vi "TakeVData_CO.vi"(0 "Sensor":u16(ring)=1 items=["No1"=1, "No 2"=2, "No 3"=3, "No 4"=4], 2 "Measurement wait time (ms)":dbl=100.0, 3 "Setpoint temperature (K)":dbl=21.72 format="%.3f", 4 "Allowable deviation (K)":dbl=0.002 format="%.4f", 5 "Number of voltage measurements\nbetween temperature check":dbl=8.0, 6 "Temperature Controller GPIB address":string="10", 8 "DMM (to sample) GPIB address":string="17", 10 "DMM2 GPIB address":string="30", 15 "Cutoff (nV)":dbl=0.3 format="%.2f") -> (7 "Mean Temp (C)":dbl=8.900000000000008e-06 format="%.6f", 9 "Temp error (C)":dbl=8.479922812684727e-07 format="%.6f", 11 "Voltage error 2 (mV)":dbl=8.479922812684727e-07 format="%.6f", 13 "Mean Voltage 2 (mV)":dbl=8.900000000000008e-06 format="%.6f", 16 "Temperature stable?":bool=TRUE, 17 "Mean Voltage 1 (mV)":dbl=2.5123402777783724e-08 format="%_4e", 18 "Voltage error 1 (mV)":dbl=9.655250545895796e-07 format="%.6f", 19 "Number of measurements":dbl=72.0)   [LabVIEW 2014]
uses:
  <vilib>/Analysis/NI_AALBase.lvlib
panel:
  out "Current mean":dbl=2.5123402777783724e-08 format="%_4e"
  out "XY Graph":T1(graph)={"X Values"=[-1.3009003499999803e-05, -9.481650499999804e-06, -5.954297499999805e-06, -2.4269444999998053e-06, 1.1004085000001942e-06, 4.627761500000194e-06, 8.155114500000194e-06, 1.1682467500000193e-05, 1.5209820500000192e-05, 1.873717350000019e-05], "Histogram: h(x)"=[6, 7, 10, 12, 13, 7, 8, 6, 1, 2]}
  out "Waveform Chart":dbl[](graph)=[-4.220760000000091e-06, -1.0250409999999939e-05, -4.8237250000000755e-06, 5.728169999999954e-06, -1.085337500000014e-05, 0.0, 8.140034999999874e-06, -3.316314999999995e-06, 5.4266849999998635e-06, -1.447117000000003e-05, -6.029655000000045e-06, -3.617790000000126e-06, -1.5074100000000805e-06, 6.934104999999904e-06, -1.3566725000000151e-05, 9.34596500000006e-06, 2.1103800000000453e-06, 1.8088999999999345e-06, -3.0148500000009085e-07, -4.522244999999965e-06, 9.34597500000002e-06, 3.014825000000141e-06, 4.522239999999985e-06, 1.2360785000000221e-05, -1.4169710000000056e-05, 1.899344000000011e-05, -4.823729999999839e-06, 9.647459999999894e-06, 8.743010000000035e-06, 0.0, -3.014800000001108e-07, -1.4772679999999804e-05, -4.220759999999874e-06, 9.34596500000006e-06, -1.2059299999999697e-06, -1.1154869999999975e-05, 6.029649999999848e-07, 1.0250424999999879e-05, 2.0500850000000192e-05, -6.331144999999682e-06, -2.71335000000001e-06, -3.014800000001108e-07, 1.1757835000000176e-05, -8.743005000000055e-06, -1.5074150000000605e-06, 6.331139999999919e-06, -2.4118649999999194e-06, 1.2059349999999497e-06, -8.140044999999834e-06, -5.728179999999914e-06, 1.5978610000000207e-05, -8.441524999999945e-06, 1.175783999999994e-05, -1.2662294999999995e-05, 9.647459999999894e-06, 1.1154869999999975e-05, -6.934115000000081e-06, -6.02964999999768e-07, -3.01484999999874e-07, -1.2059349999999497e-06, 0.0, 1.1154869999999975e-05, -3.014830000000121e-06, -7.83855999999996e-06, 5.42669500000004e-06, -3.617795000000106e-06, -3.91927999999998e-06, -1.5074150000000605e-06, 3.014830000000121e-06, -1.175783999999994e-05, -6.934115000000081e-06, 3.01484999999874e-07]
  out "Loop No.":dbl=8.0 format="%#_4f"
  out "Current precision":dbl=0.026020456598573768 format="%_6f"
  out "Current error (mV)":dbl=9.655250545895796e-07 format="%_4e"
  in  "Precision":dbl=1000.0 format="%.2f"
  # "For high precision,\n0.15 works well."
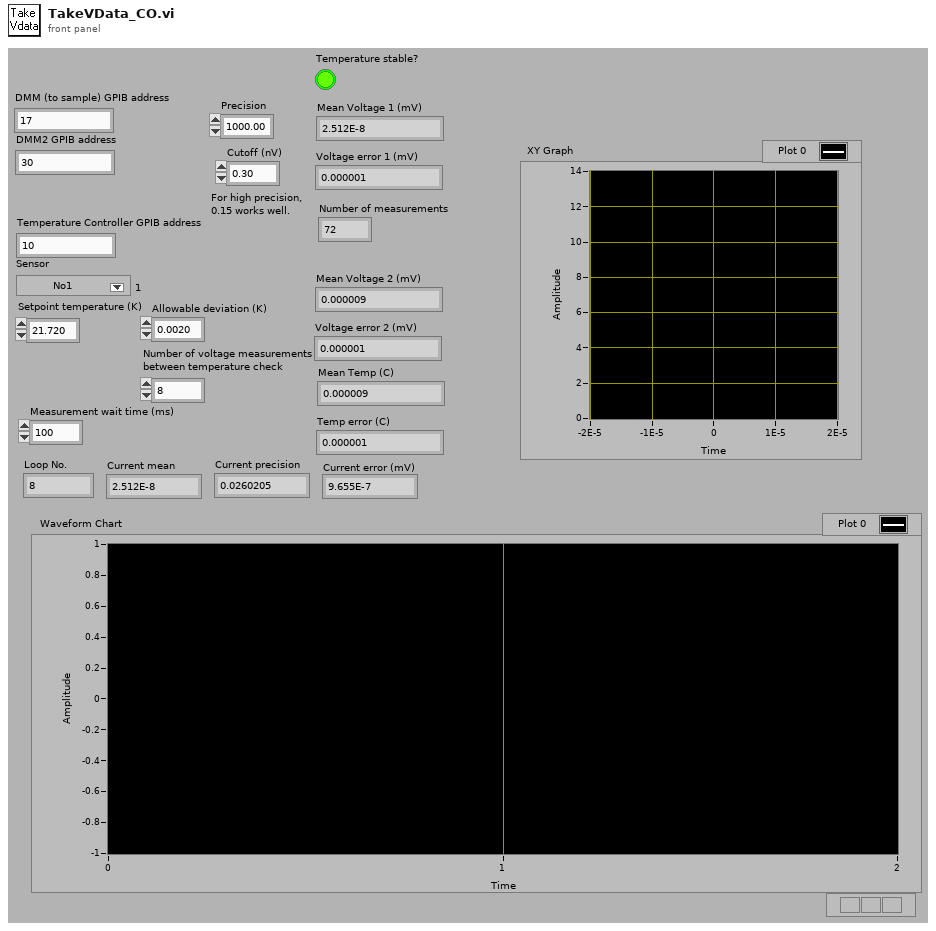
[diagram p1: front panel]
types:
  T1 = cluster{"X Values":dbl[], "Histogram: h(x)":i32[]}
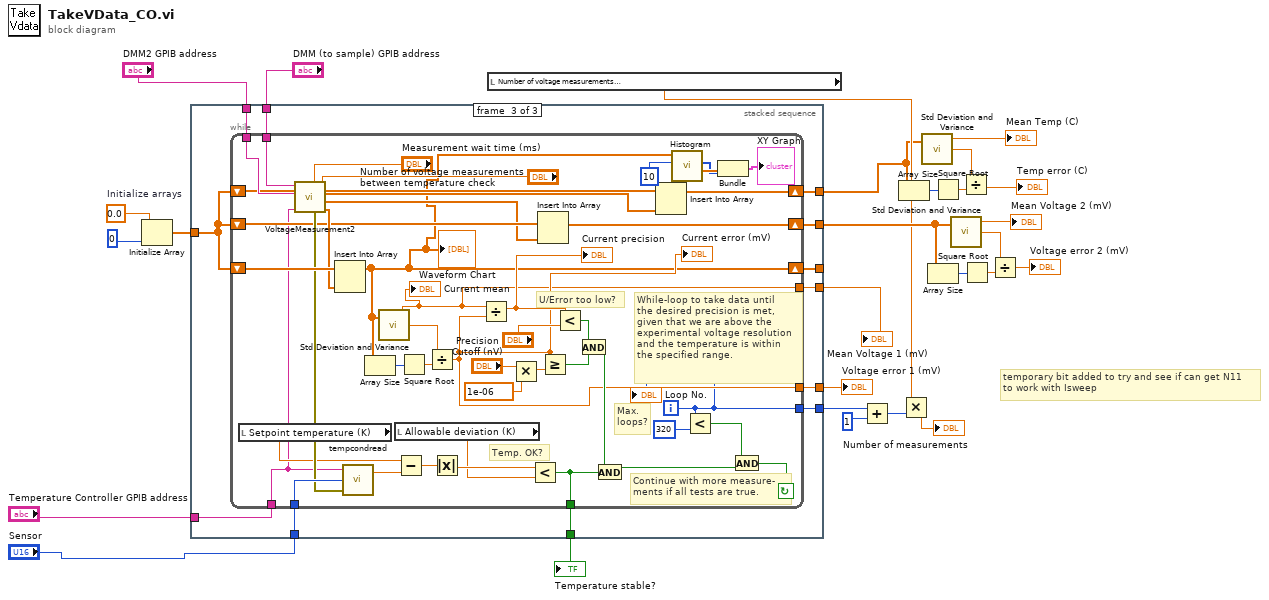
[diagram p0: block diagram]
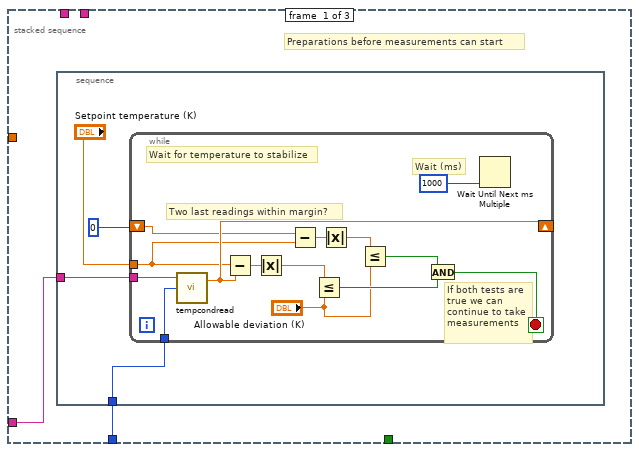
[diagram p2: hidden frame]
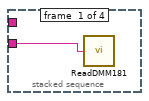
[diagram p4: hidden frame]
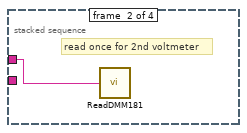
[diagram p5: hidden frame]
diagram:
  w25 = 0.0  # Initialize arrays
  # "temporary bit added to try and see if can get N11\nto work with Isweep"
  n1 = Initialize Array(w25, 0) -> (w24:dbl[])
  n2 = stacked-sequence {
    tunnel: "DMM (to sample) GPIB address" -> [_ w49 w63]
    tunnel: w24 -> [_ _ w53]
    tunnel: "Sensor" -> [w28 _ w62]
    tunnel: "Temperature Controller GPIB address" -> [w29 _ w61]
    tunnel: [_ _ w60] -> w22
    tunnel: [_ _ w59] -> _
    tunnel: [_ _ w58] -> w20
    tunnel: [_ _ w57] -> w17
    tunnel: [_ _ w56] -> w8
    tunnel: "DMM2 GPIB address" -> [_ w48 w55]
    tunnel: [_ _ w54] -> w12
    tunnel: [_ _ w52] -> w2
    frame #0 {
      # "Preparations before measurements can start"
      n3 = stacked-sequence {
        tunnel: w29 -> [w33]
        tunnel: w28 -> [w32]
        frame #0 {
          n4 = while {
            shift-left: 0 -> [w35]
            shift-right: [w37] -> _
            tunnel: w32 -> [w41]
            tunnel: w33 -> [w45]
            tunnel: "Setpoint temperature (K)" -> [w36]
            stop <- w43 stop-if-true
            # "If both tests are\ntrue we can\ncontinue to take\nmeasurements"
            # "Two last readings within margin?"
            # "Wait for temperature to stabilize"
            # "Wait (ms)"
            n5 = call "tempcondread.vi"("Ring"=w41, "GPIB Address"=w45) -> ("Temperature"=w37:dbl)  [unwired: 1 in, 1 out]
            n6 = Subtract(x=w36, y=w37) -> (x-y=w46:dbl)
            n7 = Absolute Value(x=w46) -> (abs(x)=w42:dbl)
            n8 = Subtract(x=w35, y=w36) -> (x-y=w40:dbl)
            n9 = Less Or Equal?(x=w42, y="Allowable deviation (K)") -> (x <= y?=w44:bool)
            n10 = Absolute Value(x=w40) -> (abs(x)=w39:dbl)
            n11 = Less Or Equal?(x=w39, y="Allowable deviation (K)") -> (x <= y?=w38:bool)
            n12 = And(x=w38, y=w44) -> (x .and. y?=w43:bool)
            n13 = Wait Until Next ms Multiple(millisecond multiple=1000) -> ()  [unwired: 1 out]
          }
        }
      }
    }
    frame #1 {
      n14 = stacked-sequence {
        tunnel: w49 -> [w50 _ _ _]
        tunnel: w48 -> [_ w51 _ _]
        frame #0 {
          n15 = call "ReadDMM181.vi"("DMM GPIB Address"=w50) -> ()  [unwired: 1 out]
        }
        frame #1 {
          # "read once for 2nd voltmeter"
          n16 = call "ReadDMM181.vi"("DMM GPIB Address"=w51) -> ()  [unwired: 1 out]
        }
        frame #2 {
          # "read once for 3rd voltmeter"
        }
        frame #3 {
        }
      }
    }
    frame #2 {
      n17 = while {
        shift-left: w53 -> [w79]
        shift-right: [w78] -> w52
        shift-left: w53 -> [w86]
        shift-right: [w87] -> w54
        tunnel: w55 -> [w90]
        tunnel: [w65] -> w56
        tunnel: [w72] -> w57
        tunnel: [w71] -> w58
        tunnel: [w103] -> w60
        tunnel: w61 -> [w64]
        tunnel: w62 -> [w105]
        shift-left: w53 -> [w102]
        shift-right: [w70] -> w59
        tunnel: w63 -> [w89]
        i -> [w71]
        stop <- w97 continue-if-true
        # "U/Error too low?"
        # "Max.\nloops?"
        # "Continue with more measure-\nments if all tests are true."
        # "While-loop to take data until\nthe desired precision is met,\ngiven that we are above the\nexperimental voltage resolution\nand the temperature is within\nthe specified range."
        # "Temp. OK?"
        n18 = local read "Setpoint temperature (K)"() -> (w83:dbl)
        n19 = call "VoltageMeasurement2.vi"("Number of measurements"="Number of voltage measurements\nbetween temperature check", "Measurement wait time (ms)"="Measurement wait time (ms)", "Temp Controller address"=w64, "DMM2 GPIB address"=w90, "DMM GPIB address"=w89) -> ("Voltage 1 (mV)"=w88:dbl[], "Voltage 2 (mV)"=w85:dbl[], "Voltage 3 (mV)"=w77:dbl[], "error out"=w101:errorcluster)  [unwired: 3 in]
        n20 = Insert Into Array(array=w102, new element=w88) -> (w70:dbl[])  [unwired: 1 in]
        "Waveform Chart" <- w70
        n21 = call "tempcondread.vi"("error in"=w101, "Ring"=w105, "GPIB Address"=w64) -> ("Temperature"=w106:dbl)  [unwired: 1 out]
        n22 = Array Size(array=w70) -> (size(s)=w93:i32)
        n23 = call <vilib>:"Std Deviation and Variance.vi"("X"=w70) -> ("mean"=w65:dbl, "standard deviation"=w92:dbl)  [unwired: 1 in, 1 out]
        "Current mean" <- w65
        n24 = local read "Allowable deviation (K)"() -> (w81:dbl)
        n25 = Subtract(x=w83, y=w106) -> (x-y=w107:dbl)
        n26 = Square Root(x=w93) -> (sqrt(x)=w91:dbl)
        n27 = Divide(x=w92, y=w91) -> (x/y=w72:dbl)
        "Current error (mV)" <- w72
        n28 = Absolute Value(x=w107) -> (abs(x)=w104:dbl)
        n29 = Divide(x=w65, y=w72) -> (x/y=w73:dbl)
        "Current precision" <- w73
        n30 = Multiply(x="Cutoff (nV)", y=1e-06) -> (x*y=w74:dbl)
        n31 = Less?(x=w104, y=w81) -> (x < y?=w103:bool)
        n32 = Insert Into Array(array=w86, new element=w85) -> (w87:dbl[])  [unwired: 1 in]
        n33 = Greater Or Equal?(x=w72, y=w74) -> (x >= y?=w96:bool)
        n34 = Less?(x=w73, y="Precision") -> (x < y?=w95:bool)
        n35 = And(x=w95, y=w96) -> (x .and. y?=w94:bool)
        n36 = And(x=w94, y=w103) -> (x .and. y?=w99:bool)
        n37 = Insert Into Array(array=w79, new element=w77) -> (w78:dbl[])  [unwired: 1 in]
        n38 = call <vilib>:"Histogram.vi"("intervals"=10, "X"=w70) -> ("X Values"=w67:dbl[], "Histogram: h(x)"=w66:i32[])  [unwired: 6 in, 2 out]
        n39 = Less?(x=w71, y=320) -> (x < y?=w98:bool)
        n40 = Bundle("X Values"=w67, "Histogram: h(x)"=w66) -> (→"XY Graph":T1)  [unwired: 1 in]
        n41 = And(x=w98, y=w99) -> (x .and. y?=w97:bool)
        "Loop No." <- w71
      }
    }
  }
  "Temperature stable?" <- w22
  "Voltage error 1 (mV)" <- w17
  "Mean Voltage 1 (mV)" <- w8
  n42 = local read "Number of voltage measurements\nbetween temperature check"() -> (w9:dbl)
  n43 = Add(x=w20, y=1) -> (x+y=w18:i32)
  n44 = Array Size(array=w2) -> (size(s)=w5:i32)
  n45 = Multiply(x=w9, y=w18) -> (x*y=→"Number of measurements":dbl)
  n46 = call <vilib>:"Std Deviation and Variance.vi"("X"=w2) -> ("mean"=→"Mean Temp (C)":dbl, "standard deviation"=w6:dbl)  [unwired: 1 in, 1 out]
  n47 = Array Size(array=w12) -> (size(s)=w13:i32)
  n48 = Square Root(x=w5) -> (sqrt(x)=w7:dbl)
  n49 = call <vilib>:"Std Deviation and Variance.vi"("X"=w12) -> ("mean"=→"Mean Voltage 2 (mV)":dbl, "standard deviation"=w14:dbl)  [unwired: 1 in, 1 out]
  n50 = Divide(x=w6, y=w7) -> (x/y=→"Temp error (C)":dbl)
  n51 = Square Root(x=w13) -> (sqrt(x)=w15:dbl)
  n52 = Divide(x=w14, y=w15) -> (x/y=→"Voltage error 2 (mV)":dbl)
